vi "Welcome.vi"() -> ()   [LabVIEW 2017]
uses:
  Global/Global 1.vi
  Global/Login Details.vi
  Control/WELCOM SCREEN ENUM.ctl
panel:
  out "Screen Index":i32
  in  "Check 2":bool
  in  "auto":bool
  in  "Test Print":bool
  in  "andon":bool
  in  "MANUAL":bool
  out "error out 2":errorcluster
  in  "error in (no error) 3":errorcluster
  in  "Remove":bool
  in  "Check":bool
  in  "Home":bool
  out "user name":string
  out "STOP":bool
  in  "Tab Control":enum32{"Page 1", "user mangement"}(tab)
  out "error out":errorcluster
  in  "error in (no error)":errorcluster
  in  "LOGIN":bool
  in  "RECIPE":bool
  in  "EXIT":bool
  in  "REPORT":bool
  in  "Hardware Setting":bool
  in  "Shift Setting":bool
  in  "AUTO MODE":bool
  in  "USER MANGMENT":bool
  out "datetime":string
  # "PV Clean Mobility Technologies Traceability System"
  # "USER :"
  # "Powered By - NiVision Automation Systems Pvt. Ltd."
  # "Powered By-Infinity Automation Systems Pvt Ltd. Pune"
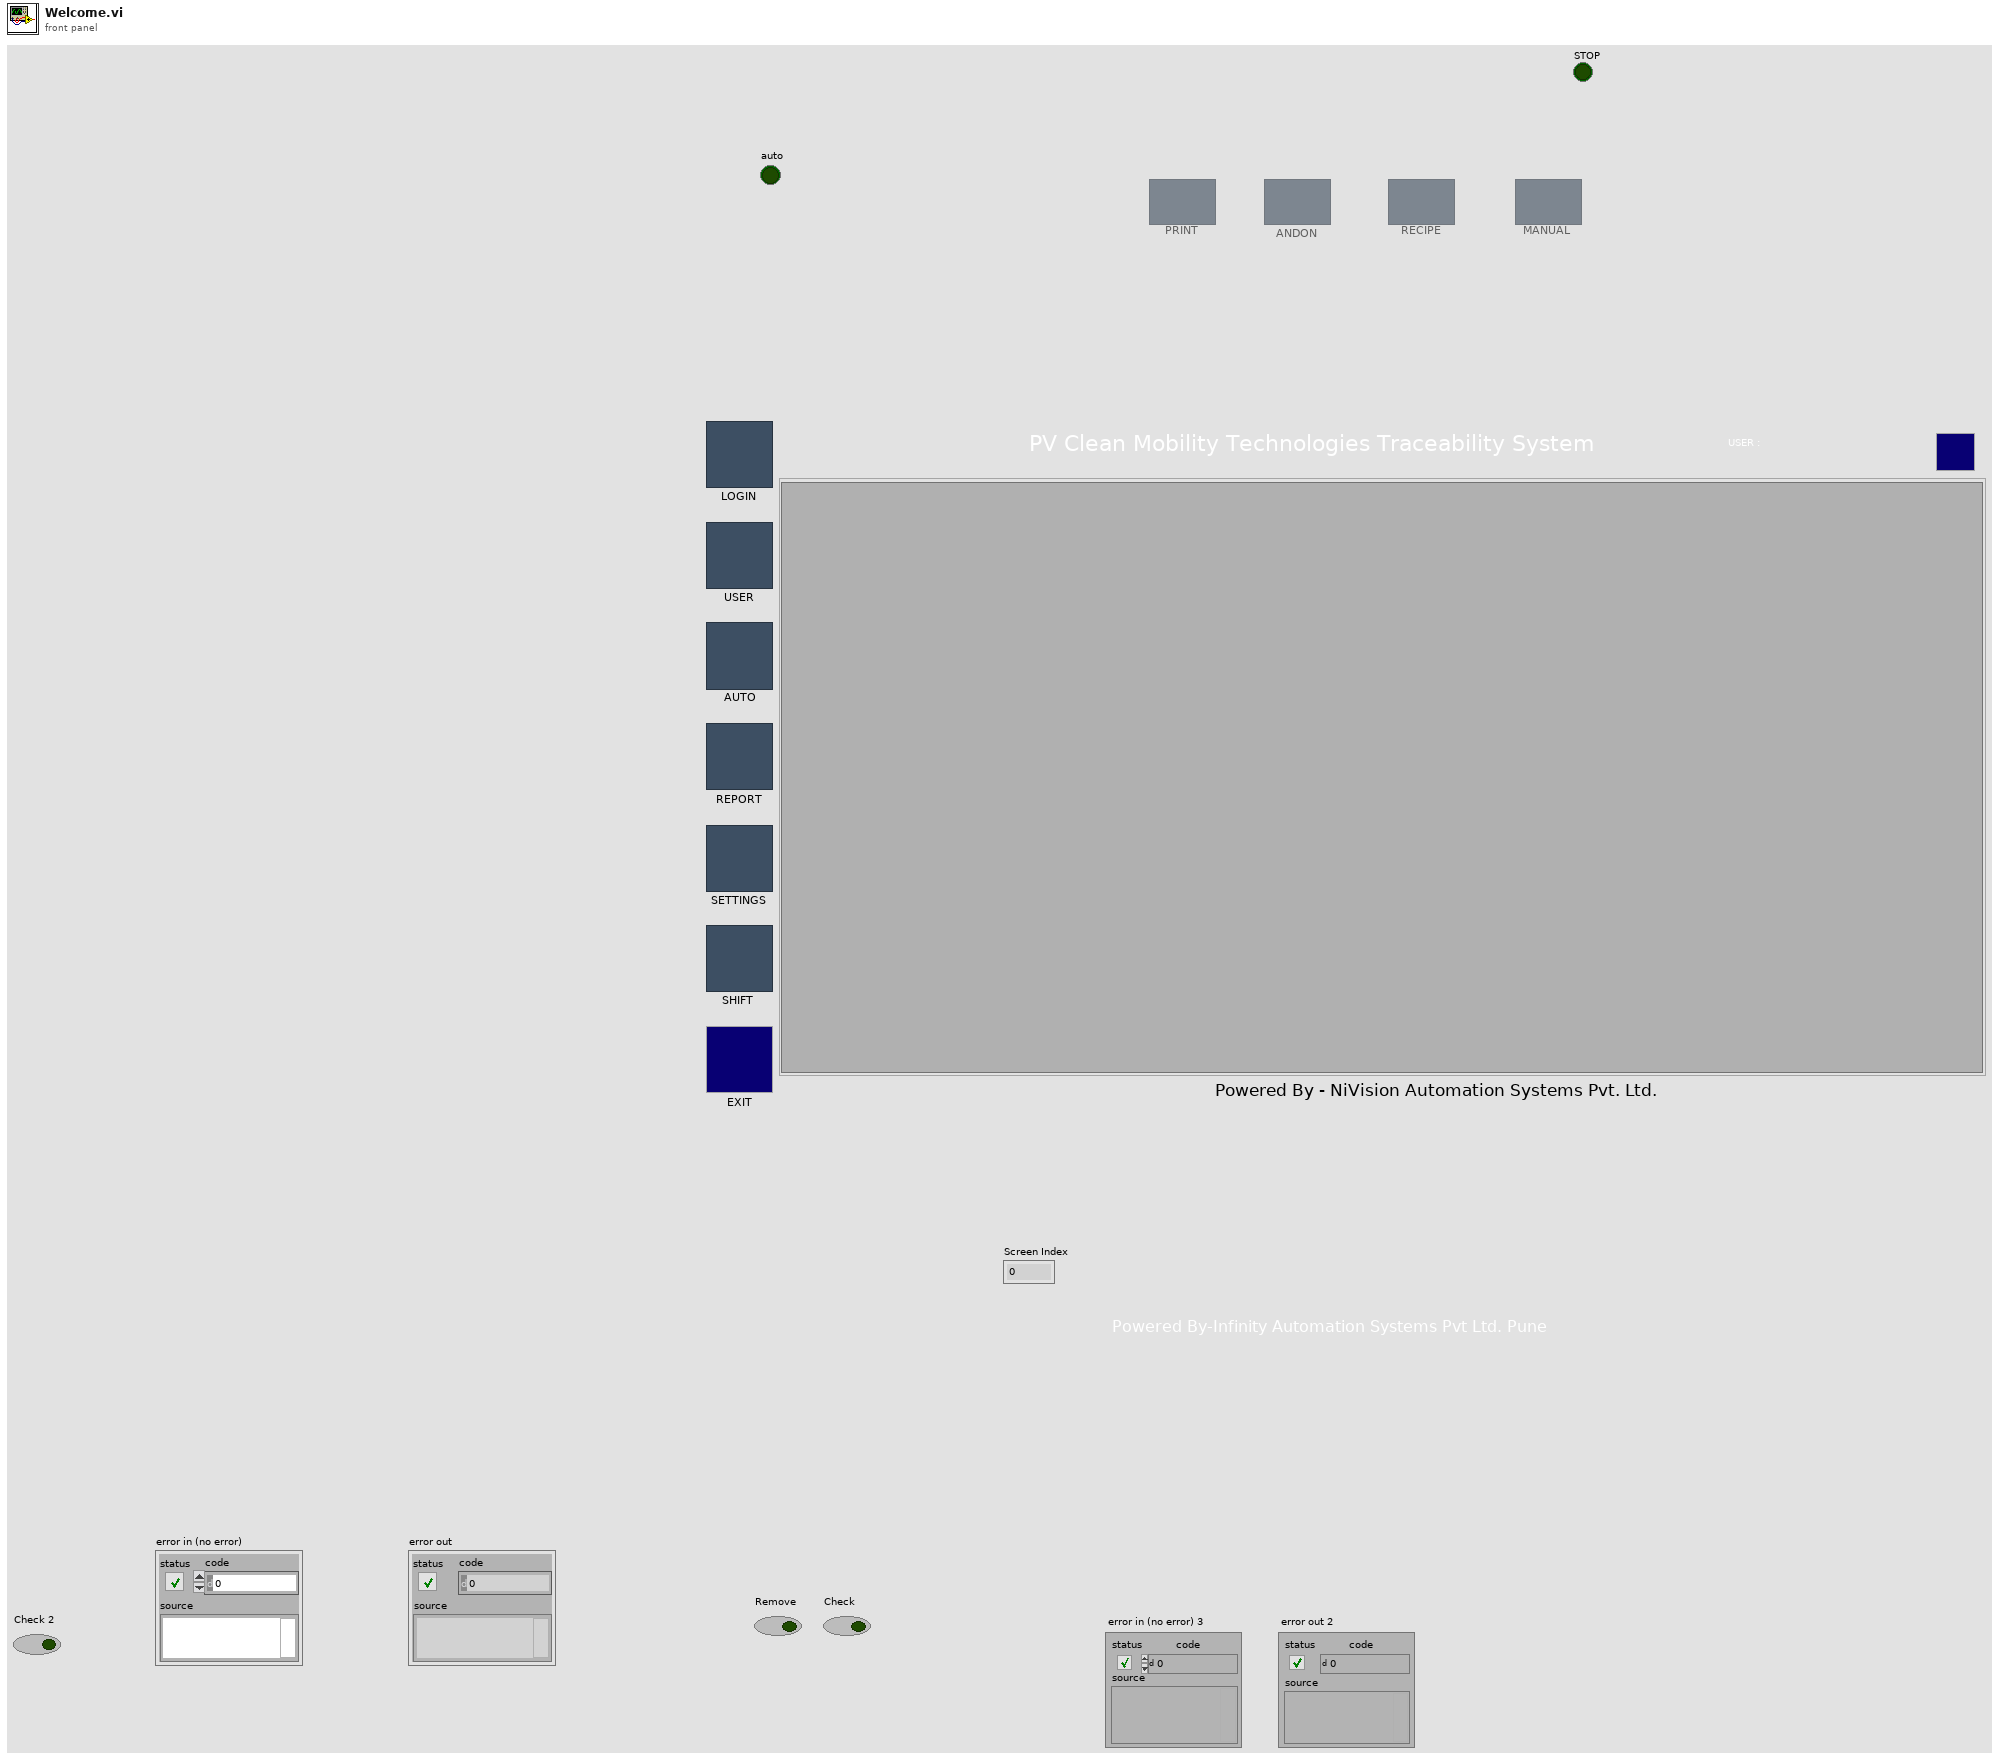
[diagram p1: front panel]
types:
  T1 = typedef "WELCOM SCREEN ENUM.ctl" = enum16{"Initialization", "Wait For Event", "RUN", "LOGIN", "USER MANAGEMENT", "AUTORITY MANAGEMENT", "AUTO MODE", "MANUAL MODE", "BIN MASTER", "CHEMICAL MASTER", "RAW MATERIAL INWARD", "RECIPE INGREDIENT", "REPORT", "SHIFT SETTING", "HARDWARE SETTING", "Check Authority", "TEST PRINT", "EXIT"}
  T2 = cluster{"SCREEN 1":bool, "SCREEN 2":bool, "SCREEN 3":bool, "SCREEN 4":bool, "SCREEN 5":bool, "SCREEN 6":bool, "SCREEN 7":bool, "SCREEN 8":bool, "SCREEN 9":bool, "SCREEN 10":bool, "SCREEN 11":bool, "SCREEN 12":bool, "SCREEN 13":bool, "SCREEN 14":bool, "SCREEN 15":bool, "SCREEN 16":bool, "SCREEN 17":bool, "SCREEN 18":bool, "SCREEN 19":bool, "SCREEN 20":bool}
  T3 = enum8{"Enabled", "Disabled", "Disabled and Grayed Out"}
  T4 = enum32{"Invalid", "Standard", "Closed", "Hidden", "Minimized", "Maximized"}
  T5 = enum32{"Bad", "Idle", "Run top level", "Running"}
  T6 = enum32{"invalid app kind", "Development System", "Run Time System", "Student Edition", "Embedded LabVIEW", "Evaluation", "Custom"}
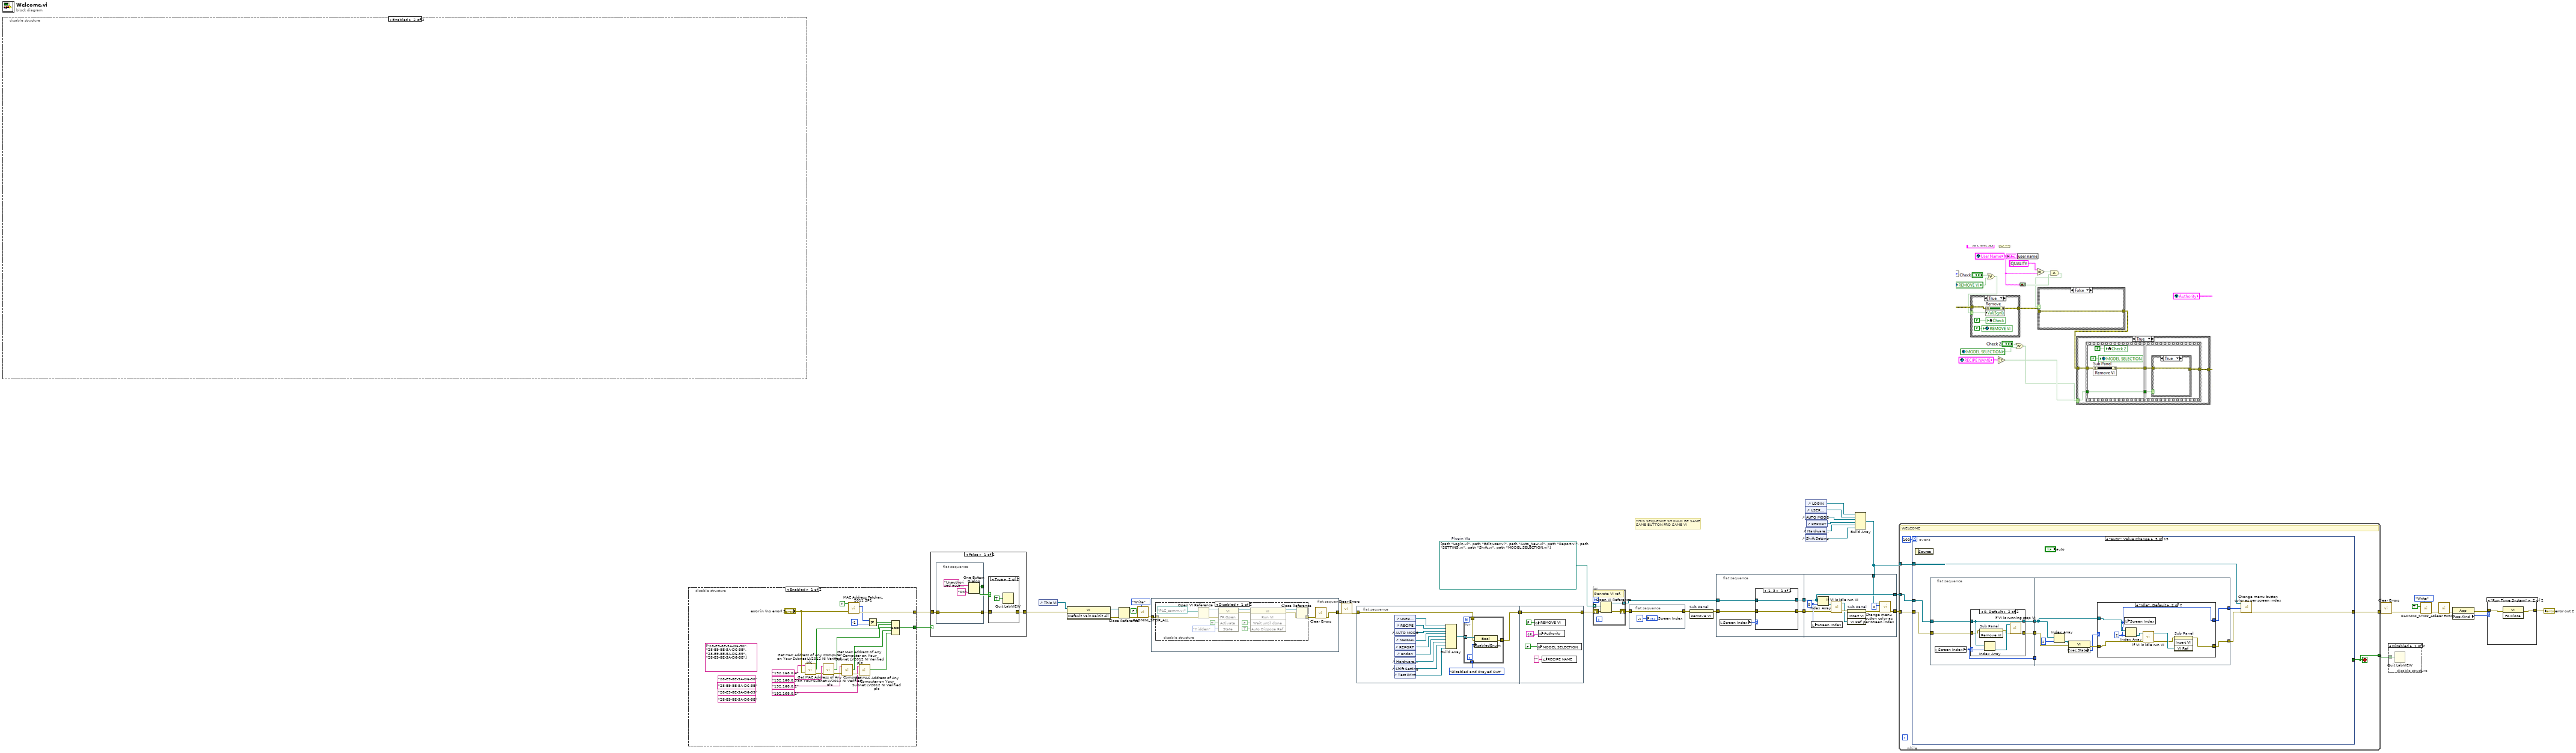
[diagram p0: block diagram]
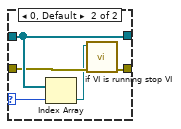
[diagram p3: hidden frame]
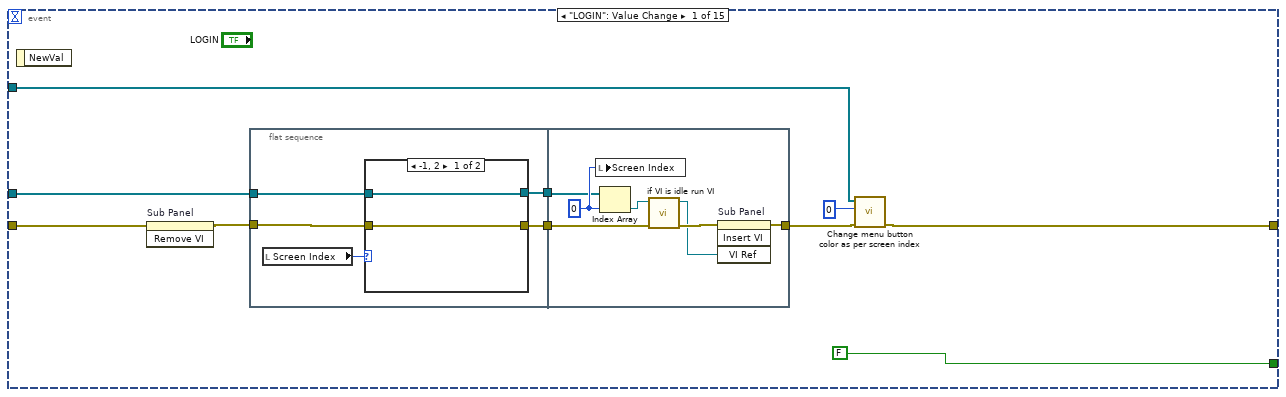
[diagram p6: hidden frame]
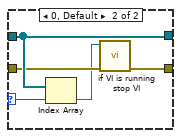
[diagram p7: hidden frame]
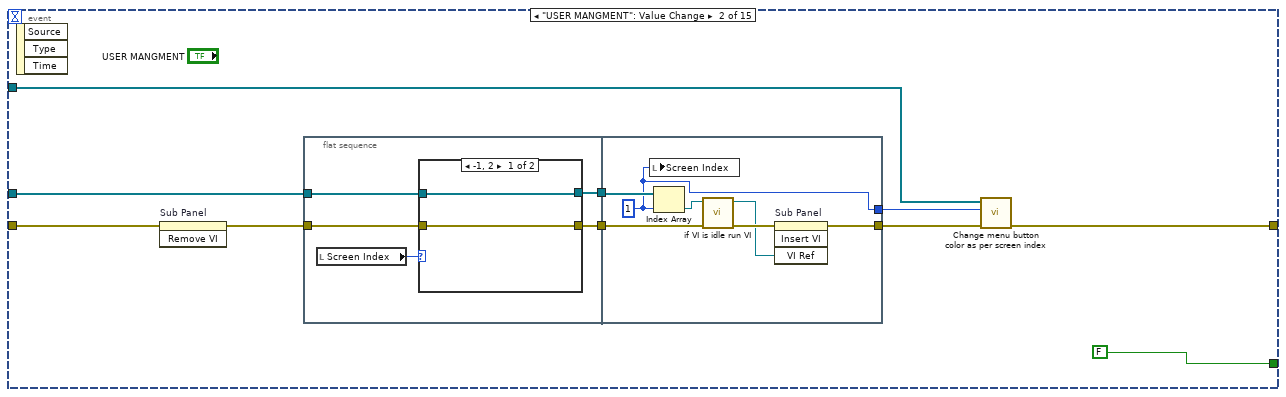
[diagram p8: hidden frame]
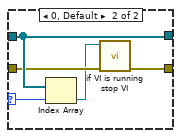
[diagram p9: hidden frame]
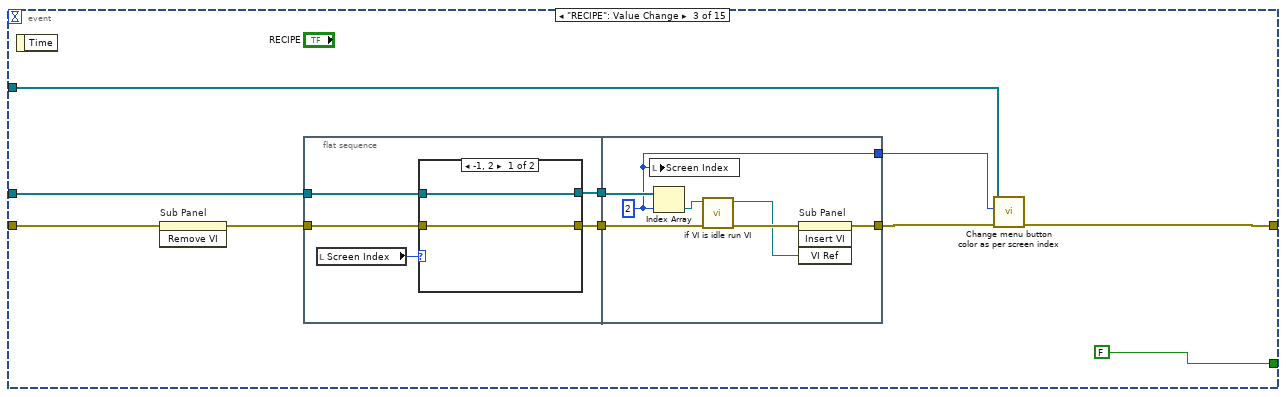
[diagram p10: hidden frame]
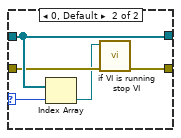
[diagram p11: hidden frame]
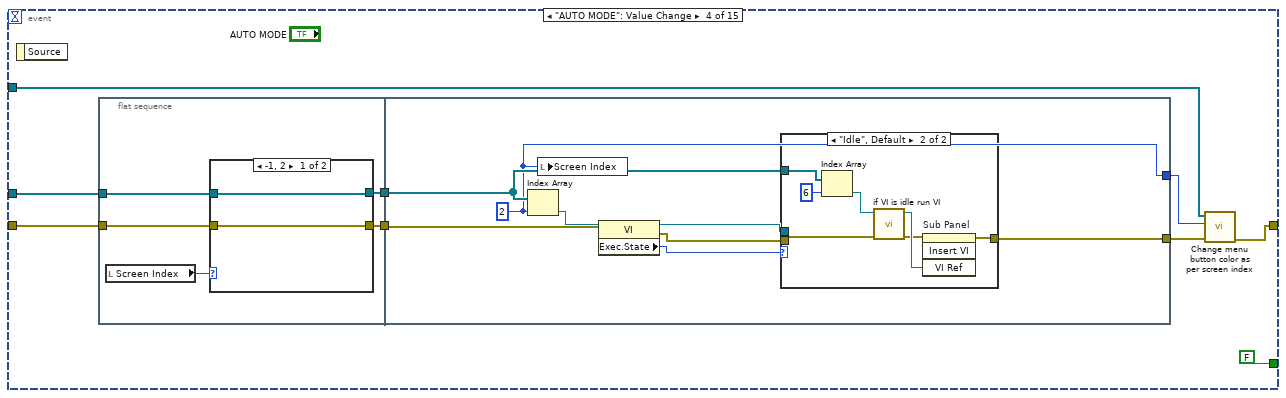
[diagram p12: hidden frame]
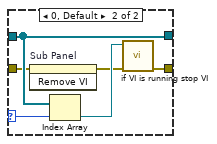
[diagram p13: hidden frame]
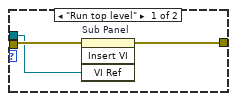
[diagram p14: hidden frame]
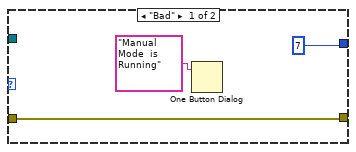
[diagram p16: hidden frame]
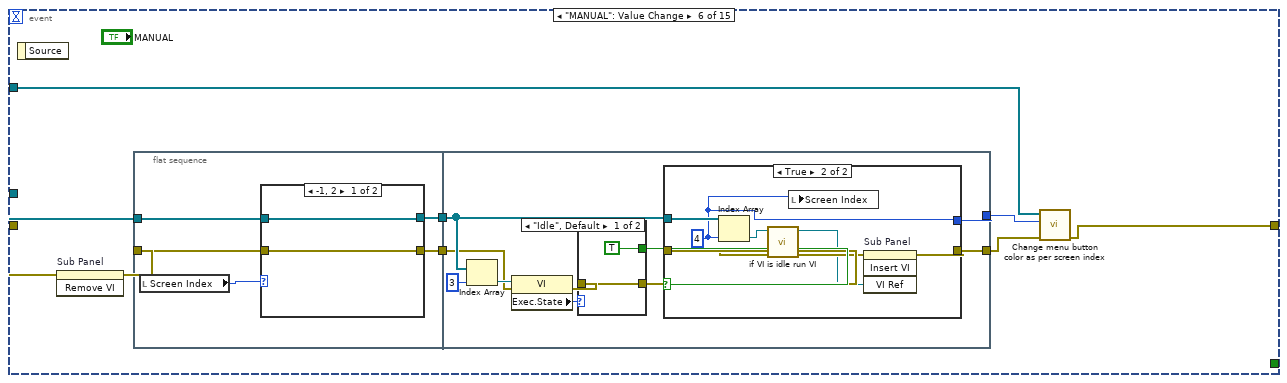
[diagram p17: hidden frame]
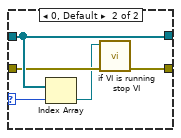
[diagram p18: hidden frame]
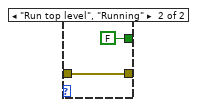
[diagram p19: hidden frame]
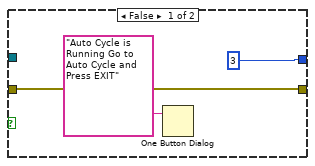
[diagram p20: hidden frame]
diagram:
  w33 = path[] [path "Login.vi", path "Edit user.vi", path "Auto_New.vi", path "Report.vi", path "SETTING.vi", path "Shift.vi", path "MODEL SELECTION.vi"]  # Plugin VIs
  # "THIS SEQUENCE SHOULD BE SAME\nSAME BUTTON FRO SAME VI"
  # "THIS SEQUENCE SHOULD BE SAME\nSAME BUTTON FRO SAME VI"
  n1 = disable-structure shown="Enabled" {
    frame Disabled {
      n2 = flat-sequence {
        tunnel: "error in (no error)" -> [w68]
        tunnel: [w67] -> w43
        frame #0 {
          n3 = invoke class="VI" method="Default Vals.Reinit All"(error in=w68) -> (error out=w67:errorcluster)  [unwired: 2 in, 2 out]
          n4 = global write "Login Details.vi" "Authority"(T2 {"SCREEN 1"=FALSE, "SCREEN 2"=FALSE, "SCREEN 3"=FALSE, "SCREEN 4"=FALSE, "SCREEN 5"=FALSE, "SCREEN 6"=FALSE, "SCREEN 7"=FALSE, "SCREEN 8"=FALSE, "SCREEN 9"=FALSE, "SCREEN 10"=FALSE, "SCREEN 11"=FALSE, "SCREEN 12"=FALSE, "SCREEN 13"=FALSE, "SCREEN 14"=FALSE, "SCREEN 15"=FALSE, "SCREEN 16"=FALSE, "SCREEN 17"=FALSE, "SCREEN 18"=FALSE, "SCREEN 19"=FALSE, "SCREEN 20"=FALSE} ("Authority")) -> ()
        }
      }
      n5 = invoke on="Sub Panel" class="SubPnl" method="Remove VI"(error in=w43) -> (error out=w56:errorcluster)  [unwired: 2 in, 2 out]
      n6 = Open VI Reference(vi path=path "Login.vi", error in (no error)=w56) -> (vi reference=w55:refnum<vi>, error out=w53:errorcluster)  [unwired: 4 in]
      n7 = invoke on="Sub Panel" class="SubPnl" method="Insert VI"(error in=w53, "VI Ref"=w55) -> (error out=w54:errorcluster)  [unwired: 2 in, 3 out]
      n8 = invoke class="VI" method="Run VI"(reference=w55, error in=w54, "Wait until done"=TRUE ("Wait Until Done"), "Auto Dispose Ref"=FALSE ("Auto Dispose Reference")) -> (reference out=w51:refnum<vi>, error out=w52:errorcluster)  [unwired: 1 in, 3 out]
      n9 = Close Reference(reference=w51, error in (no error)=w52) -> (error out=w46:errorcluster)
      n10 = Unbundle By Name(w46) -> ("code"=w50:i32)
      n11 = call <vilib>:"Clear Errors.vi"("error in (no error)"=w46) -> ("error out"=w48:errorcluster)  [unwired: 5 in, 1 out]
      n12 = Not Equal?(x=7, y=w50) -> (x != y?=w49:bool)
      n13 = Select(t=w46, s=w49, f=w48) -> (s? t:f=w47:errorcluster)
      n14 = call <vilib>:"Simple Error Handler.vi"("error in (no error)"=w47) -> ("error out"=w57:errorcluster)  [unwired: 4 in, 4 out]
      n15 = invoke on="Sub Panel" class="SubPnl" method="Remove VI"(error in=w57) -> (error out=w45:errorcluster)  [unwired: 2 in, 2 out]
      n16 = while {
        tunnel: w45 -> [w75]
        shift-right: [w77] -> _
        shift-left: WELCOM_SCREEN_ENUM."Initialization" -> [w71]
        shift-right: [w74] -> _
        shift-left: cluster{"VI Run":string} {"VI Run"=""} -> [w73]
        tunnel: [w76] -> w63
        stop <- w72 stop-if-true
        n17 = case shown="\"AUTORITY MANAGEMENT\"" w71 {
          tunnel: [WELCOM_SCREEN_ENUM."Check Authority" w102 WELCOM_SCREEN_ENUM."Wait For Event" WELCOM_SCREEN_ENUM."Wait For Event" WELCOM_SCREEN_ENUM."RUN" WELCOM_SCREEN_ENUM."RUN" WELCOM_SCREEN_ENUM."RUN" WELCOM_SCREEN_ENUM."RUN" WELCOM_SCREEN_ENUM."RUN" WELCOM_SCREEN_ENUM."RUN" WELCOM_SCREEN_ENUM."RUN" WELCOM_SCREEN_ENUM."RUN" WELCOM_SCREEN_ENUM."RUN" WELCOM_SCREEN_ENUM."RUN" WELCOM_SCREEN_ENUM."RUN" WELCOM_SCREEN_ENUM."RUN" WELCOM_SCREEN_ENUM."RUN" w229] -> w77
          tunnel: [w95 w101 w123 w127 w133 w139 w145 w151 w157 w163 w169 w175 w181 w187 w193 w199 w205 w224] -> w76
          tunnel: w75 -> [w95 w101 w123 w127 w133 w139 w145 w151 w157 w163 w169 w175 w181 w187 w193 w199 w205 w223]
          tunnel: [w93 w99 w122 w126 w131 w137 w142 w146 w155 w161 w167 w170 w177 w185 w188 w194 w203 w222] -> w74
          tunnel: w73 -> [w93 w99 w122 w126 w132 w138 w143 w147 w156 w162 w168 w171 w178 w186 w189 w195 w204 w222]
          tunnel: [FALSE FALSE FALSE TRUE FALSE FALSE FALSE FALSE FALSE FALSE FALSE FALSE FALSE FALSE FALSE FALSE FALSE FALSE] -> w72
          frame "Initialization", Default {
            n18 = control-ref of="USER MANGMENT"() -> (w80:refnum<vi>)
            n19 = control-ref of="RECIPE"() -> (w81:refnum<vi>)
            n20 = control-ref of="AUTO MODE"() -> (w82:refnum<vi>)
            n21 = control-ref of="REPORT"() -> (w88:refnum<vi>)
            n22 = control-ref of="Shift Setting"() -> (w89:refnum<vi>)
            n23 = control-ref of="Hardware Setting"() -> (w90:refnum<vi>)
            n24 = Build Array(w80, w81, w82, w88, w89, w90) -> (w79:refnum<vi>[], w83:refnum<vi>, w84:refnum<vi>, w85:refnum<vi>, w86:refnum<vi>, w87:refnum<vi>, w91:refnum<vi>)
            n25 = for {
              tunnel: w79 -> [w97] mode=indexing
              n26 = property class="Bool"(reference=w97, "DisabledEnum"=T3."Disabled and Grayed Out" ("Disabled")) -> ()  [unwired: 1 in, 2 out]
            }
          }
          frame "Wait For Event" {
            n27 = Search 1D Array(1D array=bool[] [], element=TRUE) -> (index of element=w104:i32)  [unwired: 1 in]
            n28 = case shown="11" w104 {
              tunnel: [WELCOM_SCREEN_ENUM."Wait For Event" WELCOM_SCREEN_ENUM."EXIT" WELCOM_SCREEN_ENUM."LOGIN" WELCOM_SCREEN_ENUM."USER MANAGEMENT" WELCOM_SCREEN_ENUM."AUTORITY MANAGEMENT" WELCOM_SCREEN_ENUM."AUTO MODE" WELCOM_SCREEN_ENUM."MANUAL MODE" WELCOM_SCREEN_ENUM."BIN MASTER" WELCOM_SCREEN_ENUM."CHEMICAL MASTER" WELCOM_SCREEN_ENUM."RAW MATERIAL INWARD" WELCOM_SCREEN_ENUM."REPORT" WELCOM_SCREEN_ENUM."SHIFT SETTING" WELCOM_SCREEN_ENUM."HARDWARE SETTING" WELCOM_SCREEN_ENUM."TEST PRINT" WELCOM_SCREEN_ENUM."RECIPE INGREDIENT"] -> w102
              frame -1, Default {
              }
              frame 0 {
              }
              frame 1 {
              }
              frame 2 {
              }
              frame 3 {
              }
              frame 4 {
              }
              frame 5 {
              }
              frame 6 {
              }
              frame 7 {
              }
              frame 8 {
              }
              frame 9 {
              }
              frame 10 {
              }
              frame 11 {
              }
              frame 12 {
              }
              frame 13 {
              }
            }
          }
          frame "Check Authority" {
          }
          frame "EXIT" {
          }
          frame "LOGIN" {
            w130 = "Login.vi"  # VI Run
            n29 = Bundle By Name(cluster=w132, "VI Run"=w130) -> (w131:cluster{"VI Run":string})
          }
          frame "USER MANAGEMENT" {
            w136 = "User Management.vi"  # VI Run
            n30 = Bundle By Name(cluster=w138, "VI Run"=w136) -> (w137:cluster{"VI Run":string})
          }
          frame "AUTORITY MANAGEMENT" {
            w141 = "Authority Management.vi"  # VI Run
            n31 = Bundle By Name(cluster=w143, "VI Run"=w141) -> (w142:cluster{"VI Run":string})
          }
          frame "AUTO MODE" {
            w148 = "AUTO MODE.vi"  # VI Run
            n32 = Bundle By Name(cluster=w147, "VI Run"=w148) -> (w146:cluster{"VI Run":string})
          }
          frame "MANUAL MODE" {
            w154 = "Manual Mode.vi"  # VI Run
            n33 = Bundle By Name(cluster=w156, "VI Run"=w154) -> (w155:cluster{"VI Run":string})
          }
          frame "BIN MASTER" {
            w160 = "Bin Master.vi"  # VI Run
            n34 = Bundle By Name(cluster=w162, "VI Run"=w160) -> (w161:cluster{"VI Run":string})
          }
          frame "CHEMICAL MASTER" {
            w166 = "Chemical Master.vi"  # VI Run
            n35 = Bundle By Name(cluster=w168, "VI Run"=w166) -> (w167:cluster{"VI Run":string})
          }
          frame "RAW MATERIAL INWARD" {
            w172 = "raw material inward.vi"  # VI Run
            n36 = Bundle By Name(cluster=w171, "VI Run"=w172) -> (w170:cluster{"VI Run":string})
          }
          frame "RECIPE INGREDIENT" {
            w179 = "Recipe_Ingredients.vi"  # VI Run
            n37 = Bundle By Name(cluster=w178, "VI Run"=w179) -> (w177:cluster{"VI Run":string})
          }
          frame "REPORT" {
            w184 = "Report.vi"  # VI Run
            n38 = Bundle By Name(cluster=w186, "VI Run"=w184) -> (w185:cluster{"VI Run":string})
          }
          frame "SHIFT SETTING" {
            w190 = "shift setting.vi"  # VI Run
            n39 = Bundle By Name(cluster=w189, "VI Run"=w190) -> (w188:cluster{"VI Run":string})
          }
          frame "HARDWARE SETTING" {
            w196 = "Hardware Setting.vi"  # VI Run
            n40 = Bundle By Name(cluster=w195, "VI Run"=w196) -> (w194:cluster{"VI Run":string})
          }
          frame "TEST PRINT" {
            w202 = "Test Print.vi"  # VI Run
            n41 = Bundle By Name(cluster=w204, "VI Run"=w202) -> (w203:cluster{"VI Run":string})
          }
          frame "RUN" {
            w230 = "Login.vi"  # x
            n42 = Unbundle By Name(w222) -> ("VI Run"=w231:string)
            n43 = invoke on="Sub Panel" class="SubPnl" method="Remove VI"(error in=w223) -> (error out=w212:errorcluster)  [unwired: 2 in, 2 out]
            n44 = Equal?(x=w230, y=w231) -> (x = y?=w228:bool)
            n45 = String To Path(string=w231) -> (path=w207:path)
            n46 = Open VI Reference(vi path=w207, error in (no error)=w212) -> (vi reference=w213:refnum<vi>, error out=w215:errorcluster)  [unwired: 4 in]
            n47 = invoke on="Sub Panel" class="SubPnl" method="Insert VI"(error in=w215, "VI Ref"=w213) -> (error out=w214:errorcluster)  [unwired: 2 in, 3 out]
            n48 = invoke class="VI" method="Run VI"(reference=w213, error in=w214, "Wait until done"=TRUE ("Wait Until Done"), "Auto Dispose Ref"=FALSE ("Auto Dispose Reference")) -> (reference out=w217:refnum<vi>, error out=w216:errorcluster)  [unwired: 1 in, 3 out]
            n49 = Close Reference(reference=w217, error in (no error)=w216) -> (error out=w206:errorcluster)
            n50 = Unbundle By Name(w206) -> ("code"=w218:i32)
            n51 = call <vilib>:"Clear Errors.vi"("error in (no error)"=w206) -> ("error out"=w220:errorcluster)  [unwired: 5 in, 1 out]
            n52 = Not Equal?(x=7, y=w218) -> (x != y?=w219:bool)
            n53 = Select(t=WELCOM_SCREEN_ENUM."Check Authority", s=w228, f=WELCOM_SCREEN_ENUM."Wait For Event") -> (s? t:f=w229:T1)
            n54 = Select(t=w206, s=w219, f=w220) -> (s? t:f=w221:errorcluster)
            n55 = call <vilib>:"Simple Error Handler.vi"("error in (no error)"=w221) -> ("error out"=w211:errorcluster)  [unwired: 4 in, 4 out]
            n56 = invoke on="Sub Panel" class="SubPnl" method="Remove VI"(error in=w211) -> (error out=w224:errorcluster)  [unwired: 2 in, 2 out]
          }
        }
        "STOP" <- w72
        n57 = Wait (ms)(milliseconds to wait=u32 100) -> ()  [unwired: 1 out]
      }
      n58 = while {
        tunnel: w43 -> [w65]
        tunnel: [w65] -> w41
        stop <- w66 stop-if-true
        n59 = local read "STOP"() -> (w66:bool)
      }
      n60 = Merge Errors(w41, w63) -> (→"error out":errorcluster)
      n61 = disable-structure shown="Enabled" {
        disable-tunnel: w63 -> [w70 _]
        frame Enabled {
          n62 = invoke class="VI" method="FP.Close"(error in=w70) -> ()  [unwired: 2 in, 3 out]
        }
        frame Disabled {
        }
      }
    }
    frame Enabled {
    }
  }
  n63 = disable-structure shown="Enabled" {
    disable-tunnel: [w248 _] -> w4
    disable-tunnel: [w236 TRUE] -> w2
    frame Enabled {
      (unwired) string[] ["28-E9-8E-5A-D6-50", "28-E9-8E-5A-D6-3B", "28-E9-8E-5A-D6-59", "28-E9-8E-5A-D6-5E"]
      (unwired) "28-E9-8E-5A-D6-5E" ("IP Address")
      (unwired) "28-E9-8E-5A-D6-59" ("IP Address")
      (unwired) "28-E9-8E-5A-D6-3B" ("IP Address")
      (unwired) "28-E9-8E-5A-D6-50" ("IP Address")
      n64 = call "Get MAC Address of Any Computer on Your Subnet LV2012 NI Verified plc.vi"("error constant"="error in (no error) 3", "IP Address"="192.168.0.4") -> ("error out"=w244:errorcluster, "x .and. y?"=w235:bool)  [unwired: 1 in, 1 out]
      n65 = call "Get MAC Address of Any Computer on Your Subnet LV2012 NI Verified plc.vi"("error constant"=w244, "IP Address"="192.168.0.3") -> ("error out"=w242:errorcluster, "x .and. y?"=w234:bool)  [unwired: 1 in, 1 out]
      n66 = call "Get MAC Address of Any Computer on Your Subnet LV2012 NI Verified plc.vi"("error constant"=w242, "IP Address"="192.168.0.2") -> ("error out"=w243:errorcluster, "x .and. y?"=w233:bool)  [unwired: 1 in, 1 out]
      n67 = call "MAC Address Fetcher_2011 SP1.vi"("error in (no error)"="error in (no error) 3", "Search all adapters?"=TRUE) -> ("error out"=w248:errorcluster, "index of element"=w239:i32)  [unwired: 6 in, 2 out]
      n68 = call "Get MAC Address of Any Computer on Your Subnet LV2012 NI Verified plc.vi"("error constant"=w243, "IP Address"="192.168.0.1") -> ("x .and. y?"=w232:bool)  [unwired: 1 in, 2 out]
      n69 = Not Equal?(x=w239, y=-1) -> (x != y?=w237:bool)
      n70 = Compound Arithmetic op=AND(w237, w235, w234, w233, w232) -> (w236:bool)
    }
    frame Disabled {
    }
  }
  n71 = case shown="False" w2 {
    tunnel: w4 -> [w252 w262]
    tunnel: [w251 w262] -> w3
    frame False {
      n72 = flat-sequence {
        tunnel: [w257] -> w254
        tunnel: [w256] -> w253
        tunnel: w252 -> [w256]
        frame #0 {
          n73 = One Button Dialog(message="Unauthorised access to this system\nPlease contact to NIVision Automation Systems Pvt Ltd", button name ("OK")="OK") -> (true=w257:bool)
        }
      }
      n74 = case shown="True" w254 {
        tunnel: w253 -> [w259 w260]
        tunnel: [w259 w260] -> w251
        frame False {
        }
        frame True {
          n75 = Quit LabVIEW(quit? (T)=TRUE) -> ()
        }
      }
    }
    frame True {
    }
  }
  n76 = control-ref of="This VI"() -> (w40:refnum<vi>)
  n77 = invoke class="VI" method="Default Vals.Reinit All"(reference=w40, error in=w3) -> (reference out=w38:refnum<vi>, error out=w39:errorcluster)  [unwired: 1 in, 1 out]
  n78 = Close Reference(reference=w38, error in (no error)=w39) -> (error out=w6:errorcluster)
  n79 = call "PADMINI_STOP_ALL.vi"("Enum"=enum16{"Read", "Write"}."Write", "error in (no error)"=w6, "Boolean"=FALSE) -> ("error out"=w5:errorcluster)  [unwired: 7 in, 1 out]
  n80 = flat-sequence {
    tunnel: w5 -> [w265]
    tunnel: [w263] -> w21
    frame #0 {
      n81 = disable-structure shown="Disabled" {
        disable-tunnel: w265 -> [w270 _]
        disable-tunnel: [w266 _] -> w264
        frame Disabled {
          n82 = Open VI Reference(vi path=path "PLC_comm.vi", error in (no error)=w270) -> (vi reference=w272:refnum<vi>, error out=w273:errorcluster)  [unwired: 4 in]
          n83 = invoke class="VI" method="FP.Open"(reference=w272, error in=w273, "Activate"=TRUE ("Activate?"), "State"=T4."Hidden") -> (reference out=w275:refnum<vi>, error out=w274:errorcluster)  [unwired: 1 in, 3 out]
          n84 = invoke class="VI" method="Run VI"(reference=w275, error in=w274, "Wait until done"=FALSE ("Wait Until Done"), "Auto Dispose Ref"=TRUE ("Auto Dispose Reference")) -> (reference out=w269:refnum<vi>, error out=w268:errorcluster)  [unwired: 1 in, 3 out]
          n85 = Close Reference(reference=w269, error in (no error)=w268) -> (error out=w266:errorcluster)
        }
        frame Enabled {
        }
      }
      n86 = call <vilib>:"Clear Errors.vi"("error in (no error)"=w264) -> ("error out"=w263:errorcluster)  [unwired: 5 in, 1 out]
    }
  }
  n87 = call <vilib>:"Clear Errors.vi"("error in (no error)"=w21) -> ("error out"=w20:errorcluster)  [unwired: 5 in, 1 out]
  n88 = flat-sequence {
    tunnel: w20 -> [w280]
    tunnel: [w279] -> w13
    tunnel: [w300] -> w23
    tunnel: w13 -> [w300]
    frame #0 {
      n89 = control-ref of="Shift Setting"() -> (w284:refnum<vi>)
      n90 = control-ref of="Test Print"() -> (w283:refnum<vi>)
      n91 = control-ref of="USER MANGMENT"() -> (w291:refnum<vi>)
      n92 = control-ref of="RECIPE"() -> (w290:refnum<vi>)
      n93 = control-ref of="AUTO MODE"() -> (w289:refnum<vi>)
      n94 = control-ref of="MANUAL"() -> (w288:refnum<vi>)
      n95 = control-ref of="REPORT"() -> (w287:refnum<vi>)
      n96 = control-ref of="andon"() -> (w286:refnum<vi>)
      n97 = control-ref of="Hardware Setting"() -> (w285:refnum<vi>)
      n98 = Build Array(w291, w290, w289, w288, w287, w286, w285, w284, w283) -> (w282:refnum<vi>[])
      n99 = for {
        tunnel: w282 -> [w295] mode=indexing
        tunnel: w280 -> [w294]
        tunnel: T3."Disabled and Grayed Out" ("Disabled") -> [w293]
        tunnel: [w292] -> w279
        n100 = property class="Bool"(reference=w295, error in=w294, "DisabledEnum"=w293) -> (error out=w292:errorcluster)  [unwired: 1 out]
      }
    }
    frame #1 {
      n101 = global write "Global 1.vi" "REMOVE VI"(FALSE ("REMOVE VI")) -> ()
      n102 = global write "Global 1.vi" "MODEL SELECTION"(FALSE ("REMOVE VI")) -> ()
      n103 = global write "Login Details.vi" "Authority"(T2 {"SCREEN 1"=FALSE, "SCREEN 2"=FALSE, "SCREEN 3"=FALSE, "SCREEN 4"=FALSE, "SCREEN 5"=FALSE, "SCREEN 6"=FALSE, "SCREEN 7"=FALSE, "SCREEN 8"=FALSE, "SCREEN 9"=FALSE, "SCREEN 10"=FALSE, "SCREEN 11"=FALSE, "SCREEN 12"=FALSE, "SCREEN 13"=FALSE, "SCREEN 14"=FALSE, "SCREEN 15"=FALSE, "SCREEN 16"=FALSE, "SCREEN 17"=FALSE, "SCREEN 18"=FALSE, "SCREEN 19"=FALSE, "SCREEN 20"=FALSE} ("Authority")) -> ()
      n104 = global write "Global 1.vi" "RECIPE NAME"("" ("RECIPE NAME")) -> ()
    }
  }
  n105 = for {
    tunnel: w33 -> [w302] mode=indexing
    tunnel: [w303] -> w26 mode=indexing
    shift-right: [w304] -> w32
    shift-left: w23 -> [w301]
    # "Genrate VI ref."
    n106 = Open VI Reference(vi path=w302, error in (no error)=w301) -> (vi reference=w303:refnum<vi>, error out=w304:errorcluster)  [unwired: 4 in]
  }
  n107 = flat-sequence {
    tunnel: w32 -> [w306]
    tunnel: [w306] -> w28
    frame #0 {
      "Screen Index" <- -1 ("Screen Index")
    }
  }
  n108 = invoke on="Sub Panel" class="SubPnl" method="Remove VI"(error in=w28) -> (error out=w29:errorcluster)  [unwired: 2 in, 2 out]
  n109 = flat-sequence {
    tunnel: w26 -> [w309]
    tunnel: [w311] -> w31
    tunnel: [w308] -> w30
    tunnel: w29 -> [w307]
    tunnel: w31 -> [w327]
    tunnel: w30 -> [w323]
    tunnel: [w320] -> w27
    tunnel: [w323] -> w25
    tunnel: w24 -> [w319]
    frame #0 {
      n110 = local read "Screen Index"() -> (w310:i32)
      n111 = case shown="-1, 3" w310 {
        selector: w310 -> [_ w318]
        tunnel: w307 -> [w313 w316]
        tunnel: [w313 w315] -> w311
        tunnel: w309 -> [w312 w317]
        tunnel: [w312 w317] -> w308
        frame -1, 3 {
        }
        frame 0, Default {
          n112 = Index Array(array=w317, index=w318) -> (element=w314:refnum<vi>)
          n113 = call "if VI is running stop VI.vi"("error in (no error)"=w316, "VI in"=w314) -> ("error out"=w315:errorcluster)  [unwired: 8 in, 1 out]
        }
      }
    }
    frame #1 {
      w328 = 0 ("index")
      n114 = local write "Screen Index"(w328) -> ()
      n115 = Index Array(array=w323, index=w328) -> (element=w326:refnum<vi>)
      n116 = call "if VI is idle run VI.vi"("error in (no error)"=w327, "VI in"=w326) -> ("error out"=w325:errorcluster, "VI out"=w324:refnum<vi>)  [unwired: 8 in]
      n117 = invoke on="Sub Panel" class="SubPnl" method="Insert VI"(error in=w325, "VI Ref"=w324) -> (error out=w321:errorcluster)  [unwired: 2 in, 3 out]
      n118 = call "Change menu button color as per screen index.vi"("error in (no error)"=w321, "Screen Index"=0, "Array"=w319) -> ("error out"=w320:errorcluster)  [unwired: 8 in]
    }
  }
  n119 = control-ref of="LOGIN"() -> (w19:refnum<vi>)
  n120 = control-ref of="USER MANGMENT"() -> (w18:refnum<vi>)
  n121 = control-ref of="AUTO MODE"() -> (w17:refnum<vi>)
  n122 = control-ref of="Shift Setting"() -> (w14:refnum<vi>)
  n123 = control-ref of="Hardware Setting"() -> (w15:refnum<vi>)
  n124 = control-ref of="REPORT"() -> (w16:refnum<vi>)
  n125 = Build Array(w19, w18, w17, w16, w15, w14) -> (w24:refnum<vi>[])
  n126 = while {
    tunnel: w27 -> [w331]
    tunnel: [w333] -> w22
    tunnel: w25 -> [w330]
    tunnel: w24 -> [w332]
    tunnel: [w329] -> w1
    stop <- w329 stop-if-true
    # "WELCOME"
    n127 = event shown="[4] \"auto\": Value Change" {
      selector: _ -> [_ _ _ _ _ _ _ _ _ _ _ _ _ _ _]
      dyn-events: _ -> [_ _ _ _ _ _ _ _ _ _ _ _ _ _ _]
      timeout: 100 -> [_ _ _ _ _ _ _ _ _ _ _ _ _ _ _]
      tunnel: [FALSE FALSE FALSE FALSE _ _ FALSE FALSE FALSE FALSE FALSE FALSE w699 FALSE FALSE] -> w329
      tunnel: [w337 w368 w397 w429 w462 w502 w551 w580 w609 w638 w667 w694 w698 w739 w742] -> w333
      tunnel: w330 -> [w343 w372 w401 w425 w466 w505 w555 w584 w613 w642 w671 _ w700 _ _]
      tunnel: w332 -> [w336 w366 w394 w428 w465 w503 w549 w577 w606 w636 w664 w693 w703 w737 _]
      tunnel: w331 -> [w335 w364 w393 w424 w467 w504 w547 w576 w605 w634 w663 w692 w707 w736 w754]
      event "LOGIN": Value Change {
        n128 = event-data() -> ()  [unwired: 1 in, 1 out]
        n129 = invoke on="Sub Panel" class="SubPnl" method="Remove VI"(error in=w335) -> (error out=w340:errorcluster)  [unwired: 2 in, 2 out]
        n130 = flat-sequence {
          tunnel: w343 -> [w347]
          tunnel: [w349] -> w342
          tunnel: [w346] -> w341
          tunnel: w340 -> [w345]
          tunnel: w342 -> [w361]
          tunnel: w341 -> [w362]
          tunnel: [w357] -> w338
          frame #0 {
            n131 = local read "Screen Index"() -> (w348:i32)
            n132 = case shown="-1, 2" w348 {
              selector: w348 -> [_ w356]
              tunnel: w345 -> [w351 w354]
              tunnel: [w351 w353] -> w349
              tunnel: w347 -> [w350 w355]
              tunnel: [w350 w355] -> w346
              frame -1, 2 {
              }
              frame 0, Default {
                n133 = Index Array(array=w355, index=w356) -> (element=w352:refnum<vi>)
                n134 = call "if VI is running stop VI.vi"("error in (no error)"=w354, "VI in"=w352) -> ("error out"=w353:errorcluster)  [unwired: 8 in, 1 out]
              }
            }
          }
          frame #1 {
            w363 = 0 ("index")
            n135 = local write "Screen Index"(w363) -> ()
            n136 = Index Array(array=w362, index=w363) -> (element=w360:refnum<vi>)
            n137 = call "if VI is idle run VI.vi"("error in (no error)"=w361, "VI in"=w360) -> ("error out"=w359:errorcluster, "VI out"=w358:refnum<vi>)  [unwired: 8 in]
            n138 = invoke on="Sub Panel" class="SubPnl" method="Insert VI"(error in=w359, "VI Ref"=w358) -> (error out=w357:errorcluster)  [unwired: 2 in, 3 out]
          }
        }
        n139 = call "Change menu button color as per screen index.vi"("error in (no error)"=w338, "Screen Index"=0, "Array"=w336) -> ("error out"=w337:errorcluster)  [unwired: 8 in]
      }
      event "USER MANGMENT": Value Change {
        n140 = event-data() -> ()  [unwired: 1 in, 3 out]
        n141 = invoke on="Sub Panel" class="SubPnl" method="Remove VI"(error in=w364) -> (error out=w369:errorcluster)  [unwired: 2 in, 2 out]
        n142 = flat-sequence {
          tunnel: w369 -> [w378]
          tunnel: w372 -> [w375]
          tunnel: [w377] -> w371
          tunnel: [w374] -> w370
          tunnel: [w391] -> w367
          tunnel: w371 -> [w390]
          tunnel: w370 -> [w392]
          tunnel: [w386] -> w365
          frame #0 {
            n143 = local read "Screen Index"() -> (w376:i32)
            n144 = case shown="-1, 2" w376 {
              selector: w376 -> [_ w385]
              tunnel: w378 -> [w380 w383]
              tunnel: [w380 w382] -> w377
              tunnel: w375 -> [w379 w384]
              tunnel: [w379 w384] -> w374
              frame -1, 2 {
              }
              frame 0, Default {
                n145 = Index Array(array=w384, index=w385) -> (element=w381:refnum<vi>)
                n146 = call "if VI is running stop VI.vi"("error in (no error)"=w383, "VI in"=w381) -> ("error out"=w382:errorcluster)  [unwired: 8 in, 1 out]
              }
            }
          }
          frame #1 {
            w386 = 1 ("index")
            n147 = local write "Screen Index"(w386) -> ()
            n148 = Index Array(array=w392, index=w386) -> (element=w388:refnum<vi>)
            n149 = call "if VI is idle run VI.vi"("error in (no error)"=w390, "VI in"=w388) -> ("error out"=w389:errorcluster, "VI out"=w387:refnum<vi>)  [unwired: 8 in]
            n150 = invoke on="Sub Panel" class="SubPnl" method="Insert VI"(error in=w389, "VI Ref"=w387) -> (error out=w391:errorcluster)  [unwired: 2 in, 3 out]
          }
        }
        n151 = call "Change menu button color as per screen index.vi"("error in (no error)"=w367, "Screen Index"=w365, "Array"=w366) -> ("error out"=w368:errorcluster)  [unwired: 8 in]
      }
      event "RECIPE": Value Change {
        n152 = event-data() -> ()  [unwired: 1 in, 1 out]
        n153 = invoke on="Sub Panel" class="SubPnl" method="Remove VI"(error in=w393) -> (error out=w398:errorcluster)  [unwired: 2 in, 2 out]
        n154 = flat-sequence {
          tunnel: w398 -> [w407]
          tunnel: w401 -> [w404]
          tunnel: [w406] -> w400
          tunnel: [w403] -> w399
          tunnel: [w420] -> w396
          tunnel: w400 -> [w419]
          tunnel: w399 -> [w421]
          tunnel: [w415] -> w395
          frame #0 {
            n155 = local read "Screen Index"() -> (w405:i32)
            n156 = case shown="-1, 2" w405 {
              selector: w405 -> [_ w414]
              tunnel: w407 -> [w409 w412]
              tunnel: [w409 w411] -> w406
              tunnel: w404 -> [w408 w413]
              tunnel: [w408 w413] -> w403
              frame -1, 2 {
              }
              frame 0, Default {
                n157 = Index Array(array=w413, index=w414) -> (element=w410:refnum<vi>)
                n158 = call "if VI is running stop VI.vi"("error in (no error)"=w412, "VI in"=w410) -> ("error out"=w411:errorcluster)  [unwired: 8 in, 1 out]
              }
            }
          }
          frame #1 {
            w415 = 2 ("index")
            n159 = local write "Screen Index"(w415) -> ()
            n160 = Index Array(array=w421, index=w415) -> (element=w416:refnum<vi>)
            n161 = call "if VI is idle run VI.vi"("error in (no error)"=w419, "VI in"=w416) -> ("error out"=w418:errorcluster, "VI out"=w417:refnum<vi>)  [unwired: 8 in]
            n162 = invoke on="Sub Panel" class="SubPnl" method="Insert VI"(error in=w418, "VI Ref"=w417) -> (error out=w420:errorcluster)  [unwired: 2 in, 3 out]
          }
        }
        n163 = call "Change menu button color as per screen index.vi"("error in (no error)"=w396, "Screen Index"=w395, "Array"=w394) -> ("error out"=w397:errorcluster)  [unwired: 8 in]
      }
      event "AUTO MODE": Value Change {
        n164 = event-data() -> ()  [unwired: 1 in, 1 out]
        n165 = flat-sequence {
          tunnel: w424 -> [w435]
          tunnel: w425 -> [w433]
          tunnel: [w434] -> w427
          tunnel: [w432] -> w426
          tunnel: [w448] -> w422
          tunnel: w427 -> [w451]
          tunnel: w426 -> [w450]
          tunnel: [w449] -> w423
          frame #0 {
            n166 = local read "Screen Index"() -> (w431:i32)
            n167 = case shown="-1, 2" w431 {
              selector: w431 -> [_ w443]
              tunnel: w435 -> [w437 w439]
              tunnel: [w437 w441] -> w434
              tunnel: w433 -> [w436 w442]
              tunnel: [w436 w442] -> w432
              frame -1, 2 {
              }
              frame 0, Default {
                n168 = invoke on="Sub Panel" class="SubPnl" method="Remove VI"(error in=w439) -> (error out=w438:errorcluster)  [unwired: 2 in, 2 out]
                n169 = Index Array(array=w442, index=w443) -> (element=w440:refnum<vi>)
                n170 = call "if VI is running stop VI.vi"("error in (no error)"=w438, "VI in"=w440) -> ("error out"=w441:errorcluster)  [unwired: 8 in, 1 out]
              }
            }
          }
          frame #1 {
            w449 = 2 ("index")
            n171 = Index Array(array=w450, index=w449) -> (element=w444:refnum<vi>)
            n172 = local write "Screen Index"(w449) -> ()
            n173 = property class="VI"(reference=w444, error in=w451) -> (reference out=w445:refnum<vi>, error out=w446:errorcluster, "Exec.State"=w447:T5)
            n174 = case shown="\"Idle\", Default" w447 {
              tunnel: [w454 w459] -> w448
              tunnel: w446 -> [w453 w460]
              tunnel: w445 -> [w452 _]
              tunnel: w450 -> [_ w458]
              frame "Run top level" {
                n175 = invoke on="Sub Panel" class="SubPnl" method="Insert VI"(error in=w453, "VI Ref"=w452) -> (error out=w454:errorcluster)  [unwired: 2 in, 3 out]
              }
              frame "Idle", Default {
                n176 = Index Array(array=w458, index=6) -> (element=w457:refnum<vi>)
                n177 = call "if VI is idle run VI.vi"("error in (no error)"=w460, "VI in"=w457) -> ("error out"=w455:errorcluster, "VI out"=w461:refnum<vi>)  [unwired: 8 in]
                n178 = invoke on="Sub Panel" class="SubPnl" method="Insert VI"(error in=w455, "VI Ref"=w461) -> (error out=w459:errorcluster)  [unwired: 2 in, 3 out]
              }
            }
          }
        }
        n179 = call "Change menu button color as per screen index.vi"("error in (no error)"=w422, "Screen Index"=w423, "Array"=w428) -> ("error out"=w429:errorcluster)  [unwired: 8 in]
      }
      event "auto": Value Change {
        n180 = event-data() -> ()  [unwired: 1 in, 1 out]
        n181 = flat-sequence {
          tunnel: w467 -> [w475]
          tunnel: w466 -> [w473]
          tunnel: [w474] -> w470
          tunnel: [w472] -> w469
          tunnel: [w471] -> w468
          tunnel: [w489] -> w464
          tunnel: w470 -> [w487]
          tunnel: w469 -> [w491]
          tunnel: w468 -> [_]
          tunnel: [w490] -> w463
          frame #0 {
            n182 = local read "Screen Index"() -> (w471:i32)
            n183 = case shown="0, Default" w471 {
              selector: w471 -> [_ w483]
              tunnel: w475 -> [w477 w479]
              tunnel: [w477 w481] -> w474
              tunnel: w473 -> [w476 w482]
              tunnel: [w476 w482] -> w472
              frame -1, 2 {
              }
              frame 0, Default {
                n184 = invoke on="Sub Panel" class="SubPnl" method="Remove VI"(error in=w479) -> (error out=w478:errorcluster)  [unwired: 2 in, 2 out]
                n185 = Index Array(array=w482, index=w483) -> (element=w480:refnum<vi>)
                n186 = call "if VI is running stop VI.vi"("error in (no error)"=w478, "VI in"=w480) -> ("error out"=w481:errorcluster)  [unwired: 8 in, 1 out]
              }
            }
          }
          frame #1 {
            n187 = Index Array(array=w491, index=4) -> (element=w485:refnum<vi>)
            n188 = property class="VI"(reference=w485, error in=w487) -> (error out=w486:errorcluster, "Exec.State"=w484:T5)  [unwired: 1 out]
            n189 = case shown="\"Idle\", Default" w484 {
              tunnel: w486 -> [w494 w499]
              tunnel: [w494 w496] -> w489
              tunnel: w491 -> [_ w500]
              tunnel: [7 w498] -> w490
              frame "Bad" {
                n190 = One Button Dialog(message="Manual Mode  is Running") -> ()  [unwired: 1 in, 1 out]
              }
              frame "Idle", Default {
                w498 = 2 ("index")
                n191 = local write "Screen Index"(w498) -> ()
                n192 = Index Array(array=w500, index=w498) -> (element=w501:refnum<vi>)
                n193 = call "if VI is idle run VI.vi"("error in (no error)"=w499, "VI in"=w501) -> ("error out"=w495:errorcluster, "VI out"=w497:refnum<vi>)  [unwired: 8 in]
                n194 = invoke on="Sub Panel" class="SubPnl" method="Insert VI"(error in=w495, "VI Ref"=w497) -> (error out=w496:errorcluster)  [unwired: 2 in, 3 out]
              }
            }
          }
        }
        n195 = call "Change menu button color as per screen index.vi"("error in (no error)"=w464, "Screen Index"=w463, "Array"=w465) -> ("error out"=w462:errorcluster)  [unwired: 8 in]
      }
      event "MANUAL": Value Change {
        n196 = event-data() -> ()  [unwired: 1 in, 1 out]
        n197 = invoke on="Sub Panel" class="SubPnl" method="Remove VI"(error in=w504) -> (error out=w508:errorcluster)  [unwired: 2 in, 2 out]
        n198 = flat-sequence {
          tunnel: w508 -> [w515]
          tunnel: w505 -> [w513]
          tunnel: [w514] -> w510
          tunnel: [w512] -> w509
          tunnel: [w532] -> w507
          tunnel: w510 -> [w524]
          tunnel: w509 -> [w530]
          tunnel: [w531] -> w506
          frame #0 {
            n199 = local read "Screen Index"() -> (w511:i32)
            n200 = case shown="-1, 2" w511 {
              selector: w511 -> [_ w522]
              tunnel: w515 -> [w517 w520]
              tunnel: [w517 w519] -> w514
              tunnel: w513 -> [w516 w521]
              tunnel: [w516 w521] -> w512
              frame -1, 2 {
              }
              frame 0, Default {
                n201 = Index Array(array=w521, index=w522) -> (element=w518:refnum<vi>)
                n202 = call "if VI is running stop VI.vi"("error in (no error)"=w520, "VI in"=w518) -> ("error out"=w519:errorcluster)  [unwired: 8 in, 1 out]
              }
            }
          }
          frame #1 {
            n203 = Index Array(array=w530, index=3) -> (element=w525:refnum<vi>)
            n204 = property class="VI"(reference=w525, error in=w524) -> (error out=w528:errorcluster, "Exec.State"=w527:T5)  [unwired: 1 out]
            n205 = case shown="\"Idle\", Default" w527 {
              tunnel: w528 -> [w533 w535]
              tunnel: [TRUE FALSE] -> w526
              tunnel: [w533 w535] -> w523
              frame "Idle", Default {
              }
              frame "Run top level", "Running" {
              }
            }
            n206 = case shown="True" w526 {
              tunnel: w530 -> [_ w546]
              tunnel: [w538 w545] -> w532
              tunnel: w523 -> [w538 w544]
              tunnel: [3 ("index") w540] -> w531
              frame False {
                n207 = One Button Dialog(message="Auto Cycle is Running Go to Auto Cycle and Press EXIT") -> ()  [unwired: 1 in, 1 out]
              }
              frame True {
                w540 = 4 ("index")
                n208 = Index Array(array=w546, index=w540) -> (element=w541:refnum<vi>)
                n209 = call "if VI is idle run VI.vi"("error in (no error)"=w544, "VI in"=w541) -> ("error out"=w543:errorcluster, "VI out"=w542:refnum<vi>)  [unwired: 8 in]
                n210 = local write "Screen Index"(w540) -> ()
                n211 = invoke on="Sub Panel" class="SubPnl" method="Insert VI"(error in=w543, "VI Ref"=w542) -> (error out=w545:errorcluster)  [unwired: 2 in, 3 out]
              }
            }
          }
        }
        n212 = call "Change menu button color as per screen index.vi"("error in (no error)"=w507, "Screen Index"=w506, "Array"=w503) -> ("error out"=w502:errorcluster)  [unwired: 8 in]
      }
      event "REPORT": Value Change {
        n213 = event-data() -> ()  [unwired: 1 in, 3 out]
        n214 = invoke on="Sub Panel" class="SubPnl" method="Remove VI"(error in=w547) -> (error out=w552:errorcluster)  [unwired: 2 in, 2 out]
        n215 = flat-sequence {
          tunnel: w552 -> [w561]
          tunnel: w555 -> [w558]
          tunnel: [w560] -> w554
          tunnel: [w557] -> w553
          tunnel: [w574] -> w550
          tunnel: w554 -> [w573]
          tunnel: w553 -> [w575]
          tunnel: [w569] -> w548
          frame #0 {
            n216 = local read "Screen Index"() -> (w559:i32)
            n217 = case shown="-1, 2" w559 {
              selector: w559 -> [_ w568]
              tunnel: w561 -> [w563 w566]
              tunnel: [w563 w565] -> w560
              tunnel: w558 -> [w562 w567]
              tunnel: [w562 w567] -> w557
              frame -1, 2 {
              }
              frame 0, Default {
                n218 = Index Array(array=w567, index=w568) -> (element=w564:refnum<vi>)
                n219 = call "if VI is running stop VI.vi"("error in (no error)"=w566, "VI in"=w564) -> ("error out"=w565:errorcluster)  [unwired: 8 in, 1 out]
              }
            }
          }
          frame #1 {
            w569 = 3 ("index")
            n220 = local write "Screen Index"(w569) -> ()
            n221 = Index Array(array=w575, index=w569) -> (element=w570:refnum<vi>)
            n222 = call "if VI is idle run VI.vi"("error in (no error)"=w573, "VI in"=w570) -> ("error out"=w572:errorcluster, "VI out"=w571:refnum<vi>)  [unwired: 8 in]
            n223 = invoke on="Sub Panel" class="SubPnl" method="Insert VI"(error in=w572, "VI Ref"=w571) -> (error out=w574:errorcluster)  [unwired: 2 in, 3 out]
          }
        }
        n224 = call "Change menu button color as per screen index.vi"("error in (no error)"=w550, "Screen Index"=w548, "Array"=w549) -> ("error out"=w551:errorcluster)  [unwired: 8 in]
      }
      event "andon": Value Change {
        n225 = event-data() -> ()  [unwired: 1 in, 3 out]
        n226 = invoke on="Sub Panel" class="SubPnl" method="Remove VI"(error in=w576) -> (error out=w581:errorcluster)  [unwired: 2 in, 2 out]
        n227 = flat-sequence {
          tunnel: w581 -> [w590]
          tunnel: w584 -> [w587]
          tunnel: [w589] -> w583
          tunnel: [w586] -> w582
          tunnel: [w603] -> w579
          tunnel: w583 -> [w602]
          tunnel: w582 -> [w604]
          tunnel: [w598] -> w578
          frame #0 {
            n228 = local read "Screen Index"() -> (w588:i32)
            n229 = case shown="-1, 2" w588 {
              selector: w588 -> [_ w597]
              tunnel: w590 -> [w592 w595]
              tunnel: [w592 w594] -> w589
              tunnel: w587 -> [w591 w596]
              tunnel: [w591 w596] -> w586
              frame -1, 2 {
              }
              frame 0, Default {
                n230 = Index Array(array=w596, index=w597) -> (element=w593:refnum<vi>)
                n231 = call "if VI is running stop VI.vi"("error in (no error)"=w595, "VI in"=w593) -> ("error out"=w594:errorcluster)  [unwired: 8 in, 1 out]
              }
            }
          }
          frame #1 {
            w598 = 6 ("index")
            n232 = local write "Screen Index"(w598) -> ()
            n233 = Index Array(array=w604, index=w598) -> (element=w599:refnum<vi>)
            n234 = call "if VI is idle run VI.vi"("error in (no error)"=w602, "VI in"=w599) -> ("error out"=w601:errorcluster, "VI out"=w600:refnum<vi>)  [unwired: 8 in]
            n235 = invoke on="Sub Panel" class="SubPnl" method="Insert VI"(error in=w601, "VI Ref"=w600) -> (error out=w603:errorcluster)  [unwired: 2 in, 3 out]
          }
        }
        n236 = call "Change menu button color as per screen index.vi"("error in (no error)"=w579, "Screen Index"=w578, "Array"=w577) -> ("error out"=w580:errorcluster)  [unwired: 8 in]
      }
      event "Hardware Setting": Value Change {
        n237 = event-data() -> ()  [unwired: 1 in, 3 out]
        n238 = invoke on="Sub Panel" class="SubPnl" method="Remove VI"(error in=w605) -> (error out=w610:errorcluster)  [unwired: 2 in, 2 out]
        n239 = flat-sequence {
          tunnel: w610 -> [w619]
          tunnel: w613 -> [w616]
          tunnel: [w618] -> w612
          tunnel: [w615] -> w611
          tunnel: [w632] -> w608
          tunnel: w612 -> [w631]
          tunnel: w611 -> [w633]
          tunnel: [w627] -> w607
          frame #0 {
            n240 = local read "Screen Index"() -> (w617:i32)
            n241 = case shown="-1, 2" w617 {
              selector: w617 -> [_ w626]
              tunnel: w619 -> [w621 w624]
              tunnel: [w621 w623] -> w618
              tunnel: w616 -> [w620 w625]
              tunnel: [w620 w625] -> w615
              frame -1, 2 {
              }
              frame 0, Default {
                n242 = Index Array(array=w625, index=w626) -> (element=w622:refnum<vi>)
                n243 = call "if VI is running stop VI.vi"("error in (no error)"=w624, "VI in"=w622) -> ("error out"=w623:errorcluster)  [unwired: 8 in, 1 out]
              }
            }
          }
          frame #1 {
            w627 = 4 ("index")
            n244 = local write "Screen Index"(w627) -> ()
            n245 = Index Array(array=w633, index=w627) -> (element=w628:refnum<vi>)
            n246 = call "if VI is idle run VI.vi"("error in (no error)"=w631, "VI in"=w628) -> ("error out"=w630:errorcluster, "VI out"=w629:refnum<vi>)  [unwired: 8 in]
            n247 = invoke on="Sub Panel" class="SubPnl" method="Insert VI"(error in=w630, "VI Ref"=w629) -> (error out=w632:errorcluster)  [unwired: 2 in, 3 out]
          }
        }
        n248 = call "Change menu button color as per screen index.vi"("error in (no error)"=w608, "Screen Index"=w607, "Array"=w606) -> ("error out"=w609:errorcluster)  [unwired: 8 in]
      }
      event "Shift Setting": Value Change {
        n249 = event-data() -> ()  [unwired: 1 in, 3 out]
        n250 = invoke on="Sub Panel" class="SubPnl" method="Remove VI"(error in=w634) -> (error out=w639:errorcluster)  [unwired: 2 in, 2 out]
        n251 = flat-sequence {
          tunnel: w639 -> [w648]
          tunnel: w642 -> [w645]
          tunnel: [w647] -> w641
          tunnel: [w644] -> w640
          tunnel: [w661] -> w635
          tunnel: w641 -> [w660]
          tunnel: w640 -> [w662]
          tunnel: [w656] -> w637
          frame #0 {
            n252 = local read "Screen Index"() -> (w646:i32)
            n253 = case shown="-1, 2" w646 {
              selector: w646 -> [_ w655]
              tunnel: w648 -> [w650 w653]
              tunnel: [w650 w652] -> w647
              tunnel: w645 -> [w649 w654]
              tunnel: [w649 w654] -> w644
              frame -1, 2 {
              }
              frame 0, Default {
                n254 = Index Array(array=w654, index=w655) -> (element=w651:refnum<vi>)
                n255 = call "if VI is running stop VI.vi"("error in (no error)"=w653, "VI in"=w651) -> ("error out"=w652:errorcluster)  [unwired: 8 in, 1 out]
              }
            }
          }
          frame #1 {
            w656 = 5 ("index")
            n256 = local write "Screen Index"(w656) -> ()
            n257 = Index Array(array=w662, index=w656) -> (element=w657:refnum<vi>)
            n258 = call "if VI is idle run VI.vi"("error in (no error)"=w660, "VI in"=w657) -> ("error out"=w659:errorcluster, "VI out"=w658:refnum<vi>)  [unwired: 8 in]
            n259 = invoke on="Sub Panel" class="SubPnl" method="Insert VI"(error in=w659, "VI Ref"=w658) -> (error out=w661:errorcluster)  [unwired: 2 in, 3 out]
          }
        }
        n260 = call "Change menu button color as per screen index.vi"("error in (no error)"=w635, "Screen Index"=w637, "Array"=w636) -> ("error out"=w638:errorcluster)  [unwired: 8 in]
      }
      event "Test Print": Value Change {
        n261 = event-data() -> ()  [unwired: 1 in, 3 out]
        n262 = invoke on="Sub Panel" class="SubPnl" method="Remove VI"(error in=w663) -> (error out=w668:errorcluster)  [unwired: 2 in, 2 out]
        n263 = flat-sequence {
          tunnel: w668 -> [w677]
          tunnel: w671 -> [w674]
          tunnel: [w676] -> w670
          tunnel: [w673] -> w669
          tunnel: [w690] -> w666
          tunnel: w670 -> [w689]
          tunnel: w669 -> [w691]
          tunnel: [w685] -> w665
          frame #0 {
            n264 = local read "Screen Index"() -> (w675:i32)
            n265 = case shown="-1, 2" w675 {
              selector: w675 -> [_ w684]
              tunnel: w677 -> [w679 w682]
              tunnel: [w679 w681] -> w676
              tunnel: w674 -> [w678 w683]
              tunnel: [w678 w683] -> w673
              frame -1, 2 {
              }
              frame 0, Default {
                n266 = Index Array(array=w683, index=w684) -> (element=w680:refnum<vi>)
                n267 = call "if VI is running stop VI.vi"("error in (no error)"=w682, "VI in"=w680) -> ("error out"=w681:errorcluster)  [unwired: 8 in, 1 out]
              }
            }
          }
          frame #1 {
            w685 = 9 ("index")
            n268 = local write "Screen Index"(w685) -> ()
            n269 = Index Array(array=w691, index=w685) -> (element=w686:refnum<vi>)
            n270 = call "if VI is idle run VI.vi"("error in (no error)"=w689, "VI in"=w686) -> ("error out"=w688:errorcluster, "VI out"=w687:refnum<vi>)  [unwired: 8 in]
            n271 = invoke on="Sub Panel" class="SubPnl" method="Insert VI"(error in=w688, "VI Ref"=w687) -> (error out=w690:errorcluster)  [unwired: 2 in, 3 out]
          }
        }
        n272 = call "Change menu button color as per screen index.vi"("error in (no error)"=w666, "Screen Index"=w665, "Array"=w664) -> ("error out"=w667:errorcluster)  [unwired: 8 in]
      }
      event "Home": Value Change {
        n273 = event-data() -> ()  [unwired: 1 in, 3 out]
        n274 = invoke on="Sub Panel" class="SubPnl" method="Remove VI"(error in=w692) -> (error out=w695:errorcluster)  [unwired: 2 in, 2 out]
        n275 = call "Change menu button color as per screen index.vi"("error in (no error)"=w695, "Screen Index"=-1, "Array"=w693) -> ("error out"=w694:errorcluster)  [unwired: 8 in]
      }
      event "EXIT": Value Change {
        n276 = event-data() -> ()  [unwired: 1 in, 1 out]
        n277 = Index Array(array=w700, index=2) -> (element=w706:refnum<vi>)
        n278 = Build Array(w706) -> (w705:refnum<vi>[])
        n279 = for {
          tunnel: w700 -> [w729]
          tunnel: [w728] -> w708 mode=indexing
          shift-right: [w727] -> w702
          shift-left: w707 -> [w726]
          tunnel: w705 -> [w725] mode=indexing
          n280 = property class="VI"(reference=w725, error in=w726) -> (error out=w731:errorcluster, "Exec.State"=w730:T5)  [unwired: 1 out]
          n281 = case shown="\"Run top level\", \"Running\"" w730 {
            tunnel: w731 -> [w732 w734]
            tunnel: w729 -> [_ _]
            tunnel: [TRUE FALSE] -> w728
            tunnel: [w732 w734] -> w727
            frame "Idle", Default {
            }
            frame "Run top level", "Running" {
            }
          }
        }
        n282 = And Array Elements(Boolean array=w708) -> (logical AND=w704:bool)
        n283 = case shown="False" w704 {
          tunnel: [FALSE TRUE] -> w699
          tunnel: w702 -> [w713 w717]
          tunnel: [w713 w716] -> w701
          tunnel: w700 -> [_ w715]
          frame False {
            n284 = One Button Dialog(message="Auto Cycle  is Running") -> ()  [unwired: 1 in, 1 out]
          }
          frame True {
            n285 = invoke on="Sub Panel" class="SubPnl" method="Remove VI"(error in=w717) -> (error out=w718:errorcluster)  [unwired: 2 in, 2 out]
            n286 = for {
              shift-right: [w724] -> w716
              shift-left: w718 -> [w723]
              tunnel: w715 -> [w719] mode=indexing
              n287 = call "if VI is running stop VI.vi"("error in (no error)"=w723, "VI in"=w719) -> ("error out"=w722:errorcluster, "VI out"=w721:refnum<vi>)  [unwired: 8 in]
              n288 = call <vilib>:"Clear Errors.vi"("error in (no error)"=w722) -> ("error out"=w720:errorcluster)  [unwired: 5 in, 1 out]
              n289 = Close Reference(reference=w721, error in (no error)=w720) -> (error out=w724:errorcluster)
            }
          }
        }
        n290 = call "Change menu button color as per screen index.vi"("error in (no error)"=w701, "Screen Index"=-1, "Array"=w703) -> ("error out"=w698:errorcluster)  [unwired: 8 in]
      }
      event "Remove": Value Change {
        n291 = event-data() -> ()  [unwired: 1 in, 1 out]
        n292 = invoke on="Sub Panel" class="SubPnl" method="Remove VI"(error in=w736) -> (error out=w738:errorcluster)  [unwired: 2 in, 2 out]
        n293 = call "Change menu button color as per screen index.vi"("error in (no error)"=w738, "Screen Index"=-1, "Array"=w737) -> ("error out"=w739:errorcluster)  [unwired: 8 in]
      }
      event Timeout {
        n294 = event-data() -> ()  [unwired: 1 in, 1 out]
        n295 = global read "Global 1.vi" "BARCODE RECIPE"() -> (w751:string)
        n296 = global read "Global 1.vi" "MODEL SELECTION"() -> (w752:bool)
        n297 = global read "Login Details.vi" "User Name"() -> (→"user name":string)
        n298 = Format Date/Time String(time format string (%c)="%d/ %m/ %Y\n%H:%M:%S") -> (date/time string=→"datetime":string)  [unwired: 2 in]
        n299 = Empty String/Path?(string/path=w751) -> (empty?=w750:bool)
        n300 = Or(x="Check 2", y=w752) -> (x .or. y?=w756:bool)
        n301 = global read "Global 1.vi" "REMOVE VI"() -> (w753:bool)
        n302 = case shown="True" w756 {
          tunnel: w754 -> [w784 w789]
          tunnel: [w784 w788] -> w743
          tunnel: w750 -> [_ w786]
          frame False {
          }
          frame True {
            n303 = flat-sequence {
              tunnel: w789 -> [w793]
              tunnel: [w791] -> w787
              tunnel: w786 -> [w790]
              tunnel: [w790] -> w785
              tunnel: [w796] -> w788
              tunnel: w787 -> [w797]
              tunnel: w785 -> [w795]
              frame #0 {
                n304 = invoke on="Sub Panel" class="SubPnl" method="Remove VI"(error in=w793) -> (error out=w791:errorcluster)  [unwired: 2 in, 2 out]
                n305 = global write "Global 1.vi" "MODEL SELECTION"(FALSE ("remove_VI")) -> ()
                n306 = local write "Check 2"(FALSE ("Check")) -> ()
              }
              frame #1 {
                n307 = case shown="False" w795 {
                  tunnel: w797 -> [w799 w801]
                  tunnel: [w798 w801] -> w796
                  frame False {
                    n308 = property on="auto" class="Bool (strict)"(error in=w799, "Val(Sgnl)"=TRUE ("Value (Signaling)")) -> (error out=w798:errorcluster)  [unwired: 1 in, 1 out]
                  }
                  frame True {
                  }
                }
              }
            }
          }
        }
        n309 = Or(x="Check", y=w753) -> (x .or. y?=w781:bool)
        n310 = case shown="False" w781 {
          selector: w781 -> [_ w816]
          frame False {
          }
          frame True {
            n311 = global write "Global 1.vi" "REMOVE VI"(FALSE ("remove_VI")) -> ()
            n312 = property on="Remove" class="Bool (strict)"("Val(Sgnl)"=w816) -> ()  [unwired: 2 in, 2 out]
            n313 = local write "Check"(FALSE ("Check")) -> ()
          }
        }
        n314 = global read "Login Details.vi" "Authority"() -> (w777:T2)
        n315 = Unbundle By Name(w777) -> ("SCREEN 2"=w775:bool, "SCREEN 3"=w774:bool, "SCREEN 4"=w773:bool, "SCREEN 5"=w772:bool, "SCREEN 6"=w771:bool, "SCREEN 7"=w770:bool, "SCREEN 8"=w769:bool, "SCREEN 9"=w768:bool, "SCREEN 10"=w767:bool, "SCREEN 11"=w766:bool, "SCREEN 12"=w765:bool, "SCREEN 13"=w764:bool, "SCREEN 14"=w763:bool, "SCREEN 15"=w762:bool, "SCREEN 16"=w761:bool, "SCREEN 17"=w760:bool, "SCREEN 18"=w759:bool, "SCREEN 19"=w758:bool, "SCREEN 20"=w757:bool)  [unwired: 1 out]
        n316 = control-ref of="Hardware Setting"() -> (w746:refnum<vi>)
        n317 = control-ref of="Shift Setting"() -> (w745:refnum<vi>)
        n318 = control-ref of="REPORT"() -> (w747:refnum<vi>)
        n319 = control-ref of="USER MANGMENT"() -> (w749:refnum<vi>)
        n320 = control-ref of="AUTO MODE"() -> (w748:refnum<vi>)
        n321 = Build Array(w749, w748, w747, w746, w745) -> (w744:refnum<vi>[])
        n322 = Build Array(w775, w774, w773, w772, w771, w770, w769, w768, w767, w766, w765, w764, w763, w762, w761, w760, w759, w758, w757) -> (w776:bool[])
        n323 = for {
          tunnel: w776 -> [w804] mode=indexing
          tunnel: w744 -> [w805] mode=indexing
          tunnel: w743 -> [w803]
          tunnel: [w802] -> w742
          n324 = case shown="True" w804 {
            tunnel: w805 -> [w808 w812]
            tunnel: w803 -> [w807 w811]
            tunnel: [w806 w810] -> w802
            frame True {
              n325 = property class="Bool"(reference=w808, error in=w807, "DisabledEnum"=T3."Enabled" ("Disabled")) -> (error out=w806:errorcluster)  [unwired: 1 out]
            }
            frame False {
              n326 = property class="Bool"(reference=w812, error in=w811, "DisabledEnum"=T3."Disabled and Grayed Out" ("Disabled")) -> (error out=w810:errorcluster)  [unwired: 1 out]
            }
          }
        }
      }
    }
  }
  n327 = call <vilib>:"Clear Errors.vi"("error in (no error)"=w22) -> ("error out"=w12:errorcluster)  [unwired: 5 in, 1 out]
  n328 = disable-structure shown="Disabled" {
    disable-tunnel: w1 -> [w817 _]
    frame Disabled {
      n329 = Quit LabVIEW(quit? (T)=w817) -> ()
    }
    frame Enabled {
    }
  }
  n330 = call "PADMINI_STOP_ALL.vi"("Enum"=enum16{"Read", "Write"}."Write", "error in (no error)"=w12, "Boolean"=TRUE) -> ("error out"=w9:errorcluster)  [unwired: 7 in, 1 out]
  n331 = call <vilib>:"Clear Errors.vi"("error in (no error)"=w9) -> ("error out"=w35:errorcluster)  [unwired: 5 in, 1 out]
  n332 = property class="App"(error in=w35) -> (error out=w36:errorcluster, "App.Kind"=w37:T6)  [unwired: 1 in, 1 out]
  n333 = case shown="\"Run Time System\"" w37 {
    tunnel: w36 -> [w818 w820]
    tunnel: [w818 w819] -> w34
    frame Default {
    }
    frame "Run Time System" {
      n334 = invoke class="VI" method="FP.Close"(error in=w820) -> (error out=w819:errorcluster)  [unwired: 2 in, 2 out]
    }
  }
  "error out 2" <- w34
